vi "Build Right Click Menu.vi"(8 "error in (no error)":errorcluster, 9 "Return Notifier":refnum<notifier>, 10 "Menu Click Data":T1, 11 "Main Display in":refnum<class "Main Display.lvclass">) -> (0 "error out":errorcluster, 3 "Main Display out":refnum<class "Main Display.lvclass">)   [LabVIEW 2016, in "Assert API Components.lvlib" / "Assert Display.lvlib" / "Main Display.lvlib" / "Main Display.lvclass"]
doc: "Builds up a right click menu for the main multi column list box control based on where the user clicked and which asserts are currently active."
uses:
  Main Display.lvclass
  Menu Click Data.ctl
  <vilib>/Utility/miscctls.llb/LVPoint32TypeDef.ctl
  Main Display.lvclass/Main Display.ctl
  Main Display.lvlib
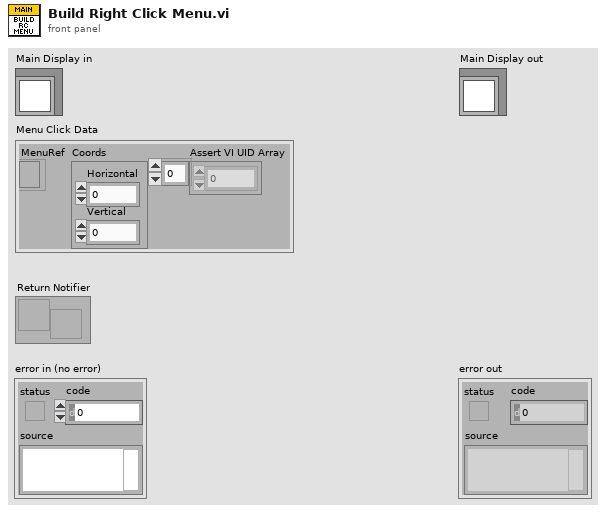
[diagram p1: front panel]
types:
  T1 = typedef "Assert API Components.lvlib/Assert Display.lvlib/Main Display.lvlib/Menu Click Data.ctl" = cluster{"MenuRef":refnum<k9>, "Coords":T2, "Assert VI UID Array":i32[]}
  T2 = typedef "LVPoint32TypeDef.ctl" = cluster{"Horizontal":i32, "Vertical":i32}
  T3 = typedef "LVRowAndColumnTypeDef.ctl" = cluster{"Row":i32, "Column":i32}
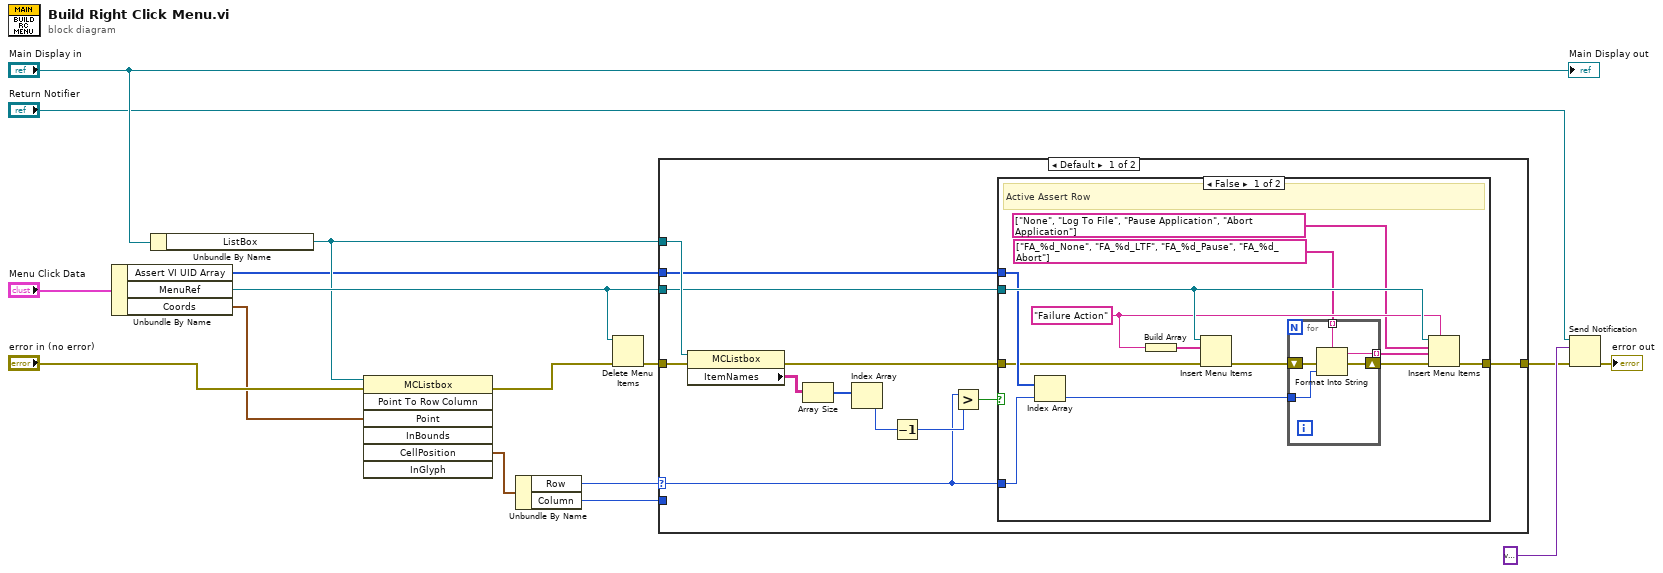
[diagram p0: block diagram]
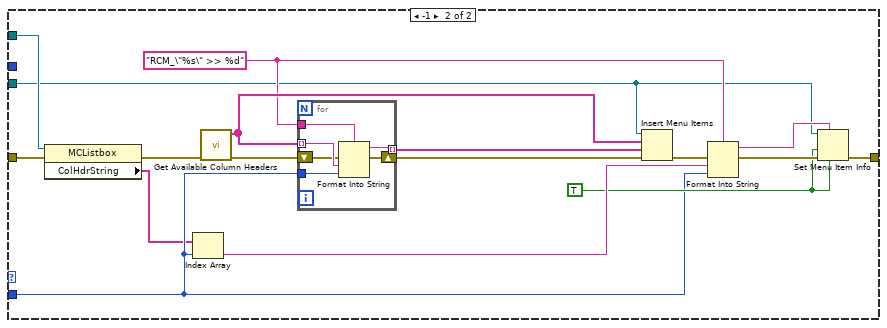
[diagram p3: hidden frame]
diagram:
  n1 = Unbundle By Name("Menu Click Data") -> ("Assert VI UID Array"=w1:i32[], "MenuRef"=w3:refnum<k9>, "Coords"=w4:T2)
  n2 = Unbundle By Name("Main Display in") -> ("ListBox"=w2:refnum<vi>)
  n3 = invoke on="Invoke Node" class="MCListbox" method="Point To Row Column"(reference=w2, error in="error in (no error)", "Point"=w4) -> (error out=w7:errorcluster, "CellPosition"=w11:T3)  [unwired: 4 in, 5 out]
  n4 = Unbundle By Name(w11) -> ("Row"=w9:i32, "Column"=w8:i32)
  n5 = Delete Menu Items(6:w7, 9:w3) -> (0:w10:errorcluster)  [unwired: 2 in, 1 out]
  n6 = case shown="Default" w9 {
    selector: w9 -> [w20 _]
    tunnel: [w18 w55] -> w5
    tunnel: w3 -> [w19 w48]
    tunnel: w10 -> [w28 w51]
    tunnel: w8 -> [_ w53]
    tunnel: w2 -> [w27 w52]
    tunnel: w1 -> [w17 _]
    frame Default {
      n7 = property class="MCListbox"(reference=w27, error in=w28) -> (error out=w21:errorcluster, "ItemNames"=w26:string[][])  [unwired: 1 out]
      n8 = Array Size(array=w26) -> (size(s)=w25:i32[])
      n9 = Index Array(array=w25) -> (element=w24:i32)  [unwired: 1 in]
      n10 = Decrement(x=w24) -> (x-1=w23:i32)
      n11 = Greater?(x=w20, y=w23) -> (0:w22:bool)
      n12 = case shown="False" w22 {
        tunnel: w21 -> [w34 w47]
        tunnel: w20 -> [w35 _]
        tunnel: w19 -> [w38 _]
        tunnel: [w39 w47] -> w18
        tunnel: w17 -> [w36 _]
        frame False {
          w37 = "Failure Action"
          # "Active Assert Row"
          n13 = Index Array(array=w36, index=w35) -> (element=w33:i32)
          n14 = Build Array(w37) -> (w40:string[])
          n15 = Insert Menu Items(6:w34, 8:w40, 9:w38) -> (0:w41:errorcluster)  [unwired: 3 in, 2 out]
          n16 = for {
            tunnel: w33 -> [w45]
            shift-right: [w44] -> w32
            shift-left: w41 -> [w46]
            tunnel: string[] ["FA_%d_None", "FA_%d_LTF", "FA_%d_Pause", "FA_%d_Abort"] -> [w43] mode=indexing
            tunnel: [w42] -> w30 mode=indexing
            n17 = Format Into String(format string=w43, error in=w46, w45) -> (resulting string=w42:string, error out=w44:errorcluster)  [unwired: 1 in]
          }
          n18 = Insert Menu Items(5:w37, 6:w32, 7:w30, 8:string[] ["None", "Log To File", "Pause Application", "Abort Application"], 9:w38) -> (0:w39:errorcluster)  [unwired: 1 in, 2 out]
        }
        frame True {
          # "Not clicked on an active assert row"
        }
      }
    }
    frame -1 {
      w54 = TRUE ("enabled")
      w59 = "RCM_\"%s\" >> %d" ("format string")
      n19 = property class="MCListbox"(reference=w52, error in=w51) -> (error out=w49:errorcluster, "ColHdrString"=w50:string[])  [unwired: 1 out]
      n20 = Index Array(array=w50, index=w53) -> (element=w58:string)
      n21 = call "Get Available Column Headers.vi"("error in (no error)"=w49) -> ("error out"=w62:errorcluster, "Available Column Headers"=w64:string[])  [unwired: 9 in]
      n22 = for {
        tunnel: w64 -> [w70] mode=indexing
        tunnel: [w69] -> w56 mode=indexing
        shift-right: [w67] -> w61
        shift-left: w62 -> [w68]
        tunnel: w59 -> [w66]
        tunnel: w53 -> [w65]
        n23 = Format Into String(format string=w66, error in=w68, w70, w65) -> (resulting string=w69:string, error out=w67:errorcluster)  [unwired: 1 in]
      }
      n24 = Insert Menu Items(6:w61, 7:w56, 8:w64, 9:w48) -> (0:w63:errorcluster)  [unwired: 2 in, 2 out]
      n25 = Format Into String(format string=w59, error in=w63, w58, w53) -> (resulting string=w57:string, error out=w60:errorcluster)  [unwired: 1 in]
      n26 = Set Menu Item Info(6:w54, 7:w57, 8:w60, 9:w54, 11:w48) -> (0:w55:errorcluster)  [unwired: 2 in, 1 out]
    }
  }
  n27 = Send Notification(notification=variant, notifier="Return Notifier", error in (no error)=w5) -> (error out=→"error out":errorcluster)  [unwired: 1 out]
  "Main Display out" <- "Main Display in"
